vi "Test_DT2_discrete.vi"() -> ()   [LabVIEW 2022 SP3]
panel:
  in  "Reset":bool
  in  "Operation":T1(ring)
  in  "f0":dbl
  in  "stop":bool
  out "Waveform Graph":dbl[][](graph)
  in  "D":dbl
  in  "Tcyc":dbl
  in  "TD":dbl
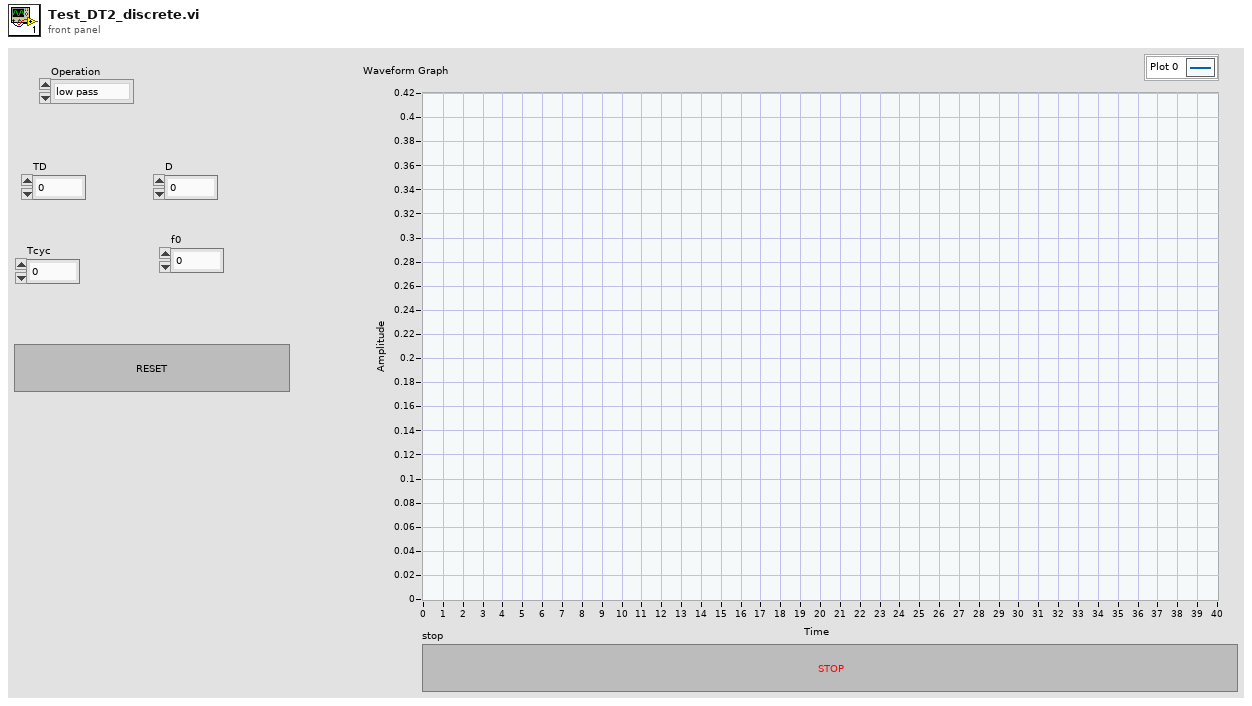
[diagram p1: front panel]
types:
  T1 = enum16{"low pass", "reset differentiation", "reset params"}
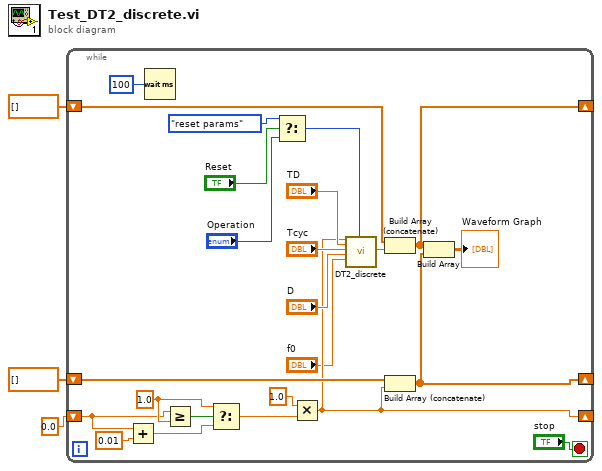
[diagram p0: block diagram]
diagram:
  n1 = while {
    shift-right: [w21] -> _
    shift-left: dbl[] [] -> [w24]
    shift-right: [w19] -> _
    shift-left: dbl[] [] -> [w23]
    shift-right: [w17] -> _
    shift-left: 0.0 -> [w11]
    stop <- "stop" stop-if-true
    w13 = 1.0 ("y")
    n2 = Add(x=w11, y=0.01) -> (x+y=w10:dbl)
    n3 = Wait (ms)(milliseconds to wait=u32 100) -> ()  [unwired: 1 out]
    n4 = Greater Or Equal?(x=w11, y=w13) -> (x >= y?=w14:bool)
    n5 = Select(t=w13, s=w14, f=w10) -> (s? t:f=w9:dbl)
    n6 = Select(t=T1."reset params" ("Operation"), s="Reset", f="Operation") -> (s? t:f=w4:T1)
    n7 = Multiply(x=1.0, y=w9) -> (x*y=w17:dbl)
    n8 = call "DT2_discrete.vi"("AI1"=w17, "TD"="TD", "Tcyc"="Tcyc", "D"="D", "f0"="f0", "Operation"=w4) -> ("AO1"=w25:dbl)  [unwired: 12 in, 1 out]
    n9 = Build Array (concatenate)(w24, w25) -> (w21:dbl[])
    n10 = Build Array (concatenate)(w23, w17) -> (w19:dbl[])
    n11 = Build Array(w21, w19) -> (→"Waveform Graph":dbl[][])
  }
